vi "add pair to buddle.vi"(5 "y":dbl, 6 "fre":dbl, 7 "x":dbl, 11 "Input":cluster{dbl[], dbl[], dbl[], dbl[]}) -> (2 "array":dbl[](array[numeric]), 3 "output":cluster{dbl[], dbl[], dbl[], dbl[]})   [LabVIEW 2021]
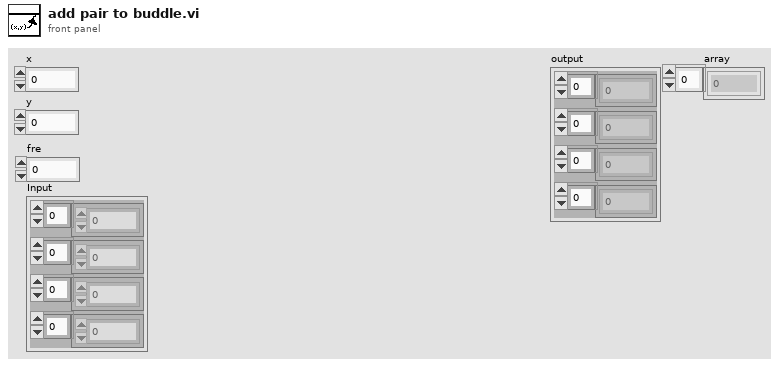
[diagram p1: front panel]
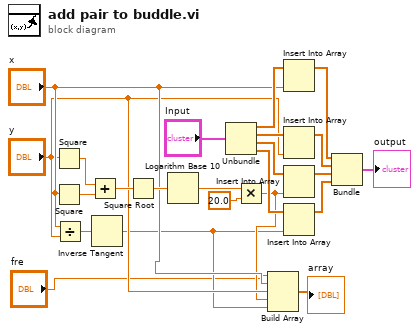
[diagram p0: block diagram]
diagram:
  n1 = Square(x="y") -> (x^2=w19:dbl)
  n2 = Square(x="x") -> (x^2=w16:dbl)
  n3 = Divide(x="x", y="y") -> (x/y=w17:dbl)
  n4 = Add(x=w19, y=w16) -> (x+y=w18:dbl)
  n5 = Inverse Tangent(1:w17) -> (0:w3:dbl)
  n6 = Square Root(x=w18) -> (sqrt(x)=w15:dbl)
  n7 = Logarithm Base 10(1:w15) -> (0:w14:dbl)
  n8 = Unbundle("Input") -> (w23:dbl[], w22:dbl[], w11:dbl[], w10:dbl[])
  n9 = Multiply(x=w14, y=20.0) -> (x*y=w4:dbl)
  n10 = Build Array("fre", "x", "y", w4, w3) -> (→"array":dbl[])
  n11 = Insert Into Array(array=w23, new element="x") -> (w21:dbl[])  [unwired: 1 in]
  n12 = Insert Into Array(array=w22, new element="y") -> (w20:dbl[])  [unwired: 1 in]
  n13 = Insert Into Array(array=w11, new element=w4) -> (w9:dbl[])  [unwired: 1 in]
  n14 = Insert Into Array(array=w10, new element=w3) -> (w8:dbl[])  [unwired: 1 in]
  n15 = Bundle(w21, w20, w9, w8) -> (→"output":cluster{dbl[], dbl[], dbl[], dbl[]})  [unwired: 1 in]
